vi "Launch Nested Task.vi"(8 "error in (no error)":errorcluster, 10 "Nested Task":refnum<class "Task.lvclass">, 11 "Task in":refnum<class "Task.lvclass">) -> (0 "error out":errorcluster, 2 "Nested EnQr":refnum<class "Message Enqueuer.lvclass">, 3 "Task out":refnum<class "Task.lvclass">)   [LabVIEW 2020, in "Volatus.lvlib" / "Task.lvclass"]
uses:
  Task.lvclass
  C:/Program Files (x86)/National Instruments/LabVIEW 2020/vi.lib/ActorFramework/Actor/Actor.lvclass
  <vilib>/ActorFramework/Message Enqueuer/Message Enqueuer.lvclass
  Task.lvclass/Task.ctl
  <vilib>/ActorFramework/Actor/Actor.lvclass
  C:/dev/lv20CE/relink/lv-volatus/Volatus/Task/Task.lvclass
  C:/dev/lv20CE/relink/lv-volatus/Volatus/APIRegistrationHandler/APIRegistrationHandler.lvclass
  C:/dev/lv20CE/relink/lv-volatus/Volatus/TaskStateHandler/TaskStateHandler.lvclass
  C:/dev/lv20CE/relink/lv-volatus/Volatus/VectoMessageHandler/VectoMessageHandler.lvclass
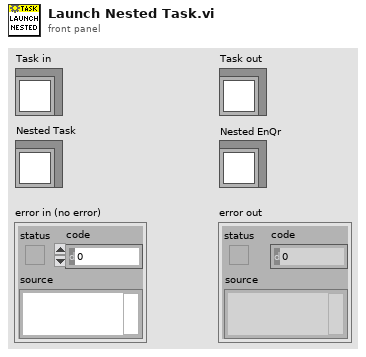
[diagram p1: front panel]
types:
  T1 = typedef "Volatus.lvlib/Core APIs.ctl" = cluster{"Volatus":refnum<class "VolatusAPI.lvclass">, "Event":refnum<class "EventAPI.lvclass">, "Telemetry":refnum<class "TelemetryAPI.lvclass">}
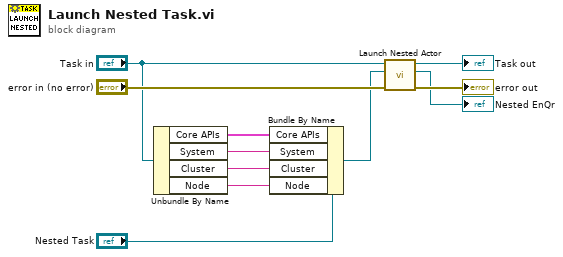
[diagram p0: block diagram]
diagram:
  n1 = Unbundle By Name("Task in") -> ("Core APIs"=w5:T1, "System"=w3:string, "Cluster"=w2:string, "Node"=w1:string)
  n2 = Bundle By Name(cluster="Nested Task", "Core APIs"=w5, "System"=w3, "Cluster"=w2, "Node"=w1) -> (w6:refnum<class "Task.lvclass">)
  n3 = call <vilib>:"Launch Nested Actor.vi"("error in (no error)"="error in (no error)", "Nested Actor"=w6, "Caller Actor in"="Task in") -> ("error out"=→"error out":errorcluster, "Nested Actor's Enqueuer"=→"Nested EnQr":refnum<class "Message Enqueuer.lvclass">, "Caller Actor out"=→"Task out":refnum<class "Task.lvclass">)  [unwired: 6 in]
